vi "VI Tree.vi"   [LabVIEW 2018, in "Keithley DMM7512.lvlib"]
doc: "This is the instrument driver for the <INSTRUMENT NAME>. The VI Tree displays all the user-callable VIs of the instrument driver in an organized table."
uses:
  <instrlib>/Keithley DMM7512/Keithley DMM7512.lvlib
panel:
  # "(c) 2015 Keithley Instruments.  ALL RIGHTS RESERVED."
  # "SEE DIAGRAM\nFOR VI TREE."
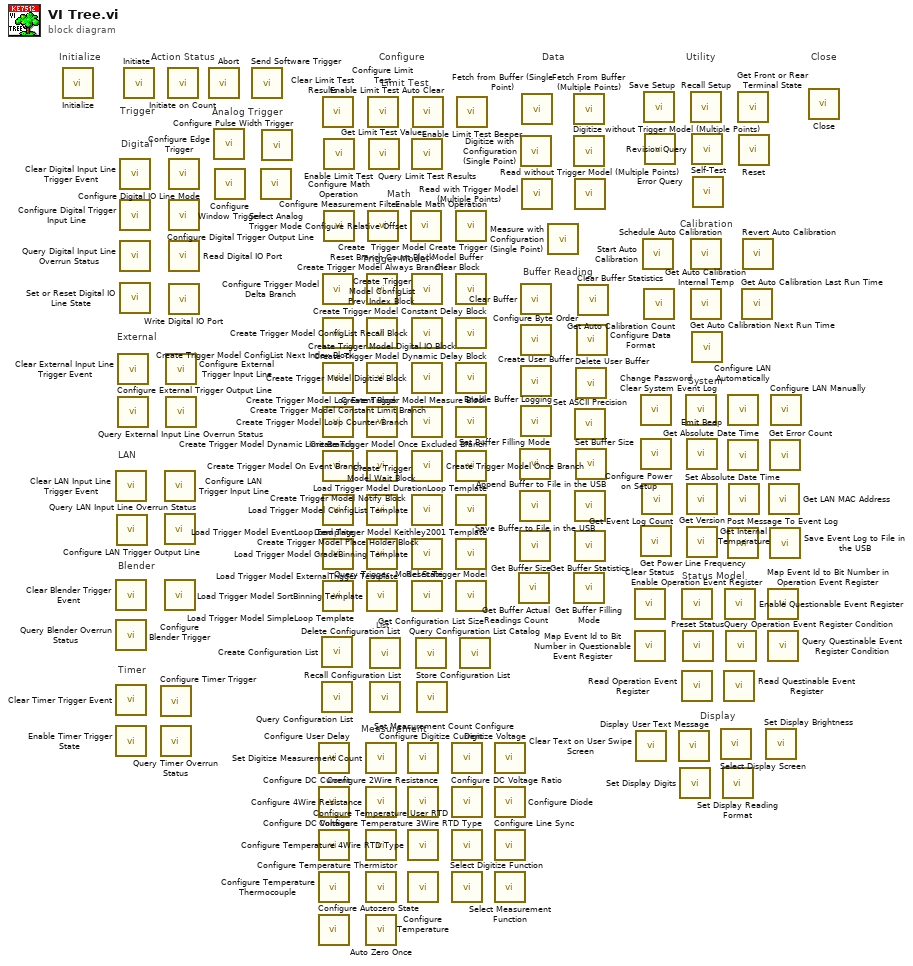
[diagram p0: block diagram]
diagram:
  # "Buffer Reading"
  # "Display"
  # "Status Model"
  # "System"
  # "Calibration"
  # "Measurement"
  # "List"
  # "Trigger Model"
  # "Math"
  # "Limit Test"
  # "Timer"
  # "Blender"
  # "LAN"
  # "External"
  # "Digital"
  # "Analog Trigger"
  # "Trigger"
  # "Action Status"
  # "Configure"
  # "Utility"
  # "Data"
  # "Close"
  # "Initialize"
  n1 = call <instrlib>:"Initialize.vi"() -> ()  [unwired: 10 in, 2 out]
  n2 = call <instrlib>:"Clear LAN Input Line Trigger Event.vi"() -> ()  [unwired: 10 in, 2 out]
  n3 = call <instrlib>:"Clear Blender Trigger Event.vi"() -> ()  [unwired: 10 in, 2 out]
  n4 = call <instrlib>:"Query Blender Overrun Status.vi"() -> ()  [unwired: 9 in, 3 out]
  n5 = call <instrlib>:"Clear Timer Trigger Event.vi"() -> ()  [unwired: 10 in, 2 out]
  n6 = call <instrlib>:"Enable Timer Trigger State.vi"() -> ()  [unwired: 14 in, 2 out]
  n7 = call <instrlib>:"Configure LAN Trigger Output Line.vi"() -> ()  [unwired: 14 in, 2 out]
  n8 = call <instrlib>:"Clear External Input Line Trigger Event.vi"() -> ()  [unwired: 10 in, 2 out]
  n9 = call <instrlib>:"Configure External Trigger Output Line.vi"() -> ()  [unwired: 10 in, 2 out]
  n10 = call <instrlib>:"Clear Digital Input Line Trigger Event.vi"() -> ()  [unwired: 10 in, 2 out]
  n11 = call <instrlib>:"Configure Digital Trigger Input Line.vi"() -> ()  [unwired: 10 in, 2 out]
  n12 = call <instrlib>:"Query Digital Input Line Overrun Status.vi"() -> ()  [unwired: 9 in, 3 out]
  n13 = call <instrlib>:"Set or Reset Digital IO Line State.vi"() -> ()  [unwired: 10 in, 2 out]
  n14 = call <instrlib>:"Initiate.vi"() -> ()  [unwired: 10 in, 2 out]
  n15 = call <instrlib>:"Configure Timer Trigger.vi"() -> ()  [unwired: 14 in, 2 out]
  n16 = call <instrlib>:"Query Timer Overrun Status.vi"() -> ()  [unwired: 9 in, 3 out]
  n17 = call <instrlib>:"Configure LAN Trigger Input Line.vi"() -> ()  [unwired: 10 in, 2 out]
  n18 = call <instrlib>:"Query LAN Input Line Overrun Status.vi"() -> ()  [unwired: 9 in, 3 out]
  n19 = call <instrlib>:"Configure Blender Trigger.vi"() -> ()  [unwired: 10 in, 2 out]
  n20 = call <instrlib>:"Configure External Trigger Input Line.vi"() -> ()  [unwired: 10 in, 2 out]
  n21 = call <instrlib>:"Query External Input Line Overrun Status.vi"() -> ()  [unwired: 9 in, 3 out]
  n22 = call <instrlib>:"Initiate on Count.vi"() -> ()  [unwired: 10 in, 2 out]
  n23 = call <instrlib>:"Configure Digital IO Line Mode.vi"() -> ()  [unwired: 10 in, 2 out]
  n24 = call <instrlib>:"Configure Digital Trigger Output Line.vi"() -> ()  [unwired: 10 in, 2 out]
  n25 = call <instrlib>:"Read Digital IO Port.vi"() -> ()  [unwired: 9 in, 3 out]
  n26 = call <instrlib>:"Write Digital IO Port.vi"() -> ()  [unwired: 10 in, 2 out]
  n27 = call <instrlib>:"Abort.vi"() -> ()  [unwired: 10 in, 2 out]
  n28 = call <instrlib>:"Configure Edge Trigger.vi"() -> ()  [unwired: 10 in, 2 out]
  n29 = call <instrlib>:"Configure Window Trigger.vi"() -> ()  [unwired: 14 in, 2 out]
  n30 = call <instrlib>:"Send Software Trigger.vi"() -> ()  [unwired: 10 in, 2 out]
  n31 = call <instrlib>:"Select Analog Trigger Mode.vi"() -> ()  [unwired: 10 in, 2 out]
  n32 = call <instrlib>:"Configure Pulse Width Trigger.vi"() -> ()  [unwired: 14 in, 2 out]
  n33 = call <instrlib>:"Configure User Delay.vi"() -> ()  [unwired: 10 in, 2 out]
  n34 = call <instrlib>:"Configure DC Current.vi"() -> ()  [unwired: 10 in, 2 out]
  n35 = call <instrlib>:"Configure DC Voltage.vi"() -> ()  [unwired: 14 in, 2 out]
  n36 = call <instrlib>:"Configure Temperature Thermocouple.vi"() -> ()  [unwired: 10 in, 2 out]
  n37 = call <instrlib>:"Configure Autozero State.vi"() -> ()  [unwired: 10 in, 2 out]
  n38 = call <instrlib>:"Create Configuration List.vi"() -> ()  [unwired: 14 in, 2 out]
  n39 = call <instrlib>:"Query Configuration List.vi"() -> ()  [unwired: 13 in, 3 out]
  n40 = call <instrlib>:"Clear Limit Test Results.vi"() -> ()  [unwired: 14 in, 2 out]
  n41 = call <instrlib>:"Configure Trigger Model Delta Branch.vi"() -> ()  [unwired: 10 in, 2 out]
  n42 = call <instrlib>:"Create Trigger Model ConfigList Next Index Block.vi"() -> ()  [unwired: 10 in, 2 out]
  n43 = call <instrlib>:"Create Trigger Model Constant Limit Branch.vi"() -> ()  [unwired: 14 in, 2 out]
  n44 = call <instrlib>:"Create Trigger Model Dynamic Limit Branch.vi"() -> ()  [unwired: 14 in, 2 out]
  n45 = call <instrlib>:"Create Trigger Model Notify Block.vi"() -> ()  [unwired: 10 in, 2 out]
  n46 = call <instrlib>:"Create Trigger Model Place Holder Block.vi"() -> ()  [unwired: 14 in, 2 out]
  n47 = call <instrlib>:"Load Trigger Model EventLoop Template.vi"() -> ()  [unwired: 14 in, 2 out]
  n48 = call <instrlib>:"Load Trigger Model SimpleLoop Template.vi"() -> ()  [unwired: 14 in, 2 out]
  n49 = call <instrlib>:"Enable Limit Test.vi"() -> ()  [unwired: 14 in, 2 out]
  n50 = call <instrlib>:"Configure Math Operation.vi"() -> ()  [unwired: 18 in, 2 out]
  n51 = call <instrlib>:"Set Digitize Measurement Count.vi"() -> ()  [unwired: 10 in, 2 out]
  n52 = call <instrlib>:"Configure 4Wire Resistance.vi"() -> ()  [unwired: 14 in, 2 out]
  n53 = call <instrlib>:"Configure Temperature User RTD.vi"() -> ()  [unwired: 10 in, 2 out]
  n54 = call <instrlib>:"Configure Temperature Thermistor.vi"() -> ()  [unwired: 10 in, 2 out]
  n55 = call <instrlib>:"Auto Zero Once.vi"() -> ()  [unwired: 10 in, 2 out]
  n56 = call <instrlib>:"Create  Trigger Model Reset Branch Count Block.vi"() -> ()  [unwired: 10 in, 2 out]
  n57 = call <instrlib>:"Create Trigger Model ConfigList Prev Index Block.vi"() -> ()  [unwired: 10 in, 2 out]
  n58 = call <instrlib>:"Create Trigger Model Digital IO Block.vi"() -> ()  [unwired: 10 in, 2 out]
  n59 = call <instrlib>:"Create Trigger Model Log Event Block.vi"() -> ()  [unwired: 10 in, 2 out]
  n60 = call <instrlib>:"Create Trigger Model On Event Branch.vi"() -> ()  [unwired: 14 in, 2 out]
  n61 = call <instrlib>:"Create Trigger Model Wait Block.vi"() -> ()  [unwired: 14 in, 2 out]
  n62 = call <instrlib>:"Load Trigger Model ExternalTrigger Template.vi"() -> ()  [unwired: 14 in, 2 out]
  n63 = call <instrlib>:"Load Trigger Model SortBinning Template.vi"() -> ()  [unwired: 26 in, 2 out]
  n64 = call <instrlib>:"Configure Limit Test.vi"() -> ()  [unwired: 14 in, 2 out]
  n65 = call <instrlib>:"Configure Measurement Filter.vi"() -> ()  [unwired: 10 in, 2 out]
  n66 = call <instrlib>:"Get Limit Test Values.vi"() -> ()  [unwired: 12 in, 4 out]
  n67 = call <instrlib>:"Delete Configuration List.vi"() -> ()  [unwired: 14 in, 2 out]
  n68 = call <instrlib>:"Recall Configuration List.vi"() -> ()  [unwired: 14 in, 2 out]
  n69 = call <instrlib>:"Set Measurement Count.vi"() -> ()  [unwired: 10 in, 2 out]
  n70 = call <instrlib>:"Configure 2Wire Resistance.vi"() -> ()  [unwired: 14 in, 2 out]
  n71 = call <instrlib>:"Configure Temperature 4Wire RTD Type.vi"() -> ()  [unwired: 10 in, 2 out]
  n72 = call <instrlib>:"Configure Temperature.vi"() -> ()  [unwired: 10 in, 2 out]
  n73 = call <instrlib>:"Configure Relative Offset.vi"() -> ()  [unwired: 10 in, 2 out]
  n74 = call <instrlib>:"Query Limit Test Results.vi"() -> ()  [unwired: 8 in, 4 out]
  n75 = call <instrlib>:"Create Trigger Model Always Branch.vi"() -> ()  [unwired: 10 in, 2 out]
  n76 = call <instrlib>:"Create Trigger Model ConfigList Recall Block.vi"() -> ()  [unwired: 10 in, 2 out]
  n77 = call <instrlib>:"Create Trigger Model Digitize Block.vi"() -> ()  [unwired: 10 in, 2 out]
  n78 = call <instrlib>:"Create Trigger Model Loop Counter Branch.vi"() -> ()  [unwired: 10 in, 2 out]
  n79 = call <instrlib>:"Create Trigger Model Once Branch.vi"() -> ()  [unwired: 10 in, 2 out]
  n80 = call <instrlib>:"Load Trigger Model ConfigList Template.vi"() -> ()  [unwired: 14 in, 2 out]
  n81 = call <instrlib>:"Load Trigger Model GradeBinning Template.vi"() -> ()  [unwired: 26 in, 2 out]
  n82 = call <instrlib>:"Query Trigger  Model State.vi"() -> ()  [unwired: 9 in, 3 out]
  n83 = call <instrlib>:"Enable Limit Test Auto Clear.vi"() -> ()  [unwired: 14 in, 2 out]
  n84 = call <instrlib>:"Get Configuration List Size.vi"() -> ()  [unwired: 13 in, 3 out]
  n85 = call <instrlib>:"Store Configuration List.vi"() -> ()  [unwired: 14 in, 2 out]
  n86 = call <instrlib>:"Configure Digitize Current.vi"() -> ()  [unwired: 14 in, 2 out]
  n87 = call <instrlib>:"Configure DC Voltage Ratio.vi"() -> ()  [unwired: 14 in, 2 out]
  n88 = call <instrlib>:"Configure Temperature 3Wire RTD Type.vi"() -> ()  [unwired: 10 in, 2 out]
  n89 = call <instrlib>:"Select Digitize Function.vi"() -> ()  [unwired: 10 in, 2 out]
  n90 = call <instrlib>:"Enable Math Operation.vi"() -> ()  [unwired: 10 in, 2 out]
  n91 = call <instrlib>:"Create Trigger Model Buffer Clear Block.vi"() -> ()  [unwired: 10 in, 2 out]
  n92 = call <instrlib>:"Create Trigger Model Constant Delay Block.vi"() -> ()  [unwired: 10 in, 2 out]
  n93 = call <instrlib>:"Create Trigger Model Dynamic Delay Block.vi"() -> ()  [unwired: 10 in, 2 out]
  n94 = call <instrlib>:"Create Trigger Model Measure Block.vi"() -> ()  [unwired: 10 in, 2 out]
  n95 = call <instrlib>:"Create Trigger Model Once Excluded Branch.vi"() -> ()  [unwired: 10 in, 2 out]
  n96 = call <instrlib>:"Load Trigger Model DurationLoop Template.vi"() -> ()  [unwired: 14 in, 2 out]
  n97 = call <instrlib>:"Load Trigger Model Keithley2001 Template.vi"() -> ()  [unwired: 14 in, 2 out]
  n98 = call <instrlib>:"Reset Trigger Model.vi"() -> ()  [unwired: 14 in, 2 out]
  n99 = call <instrlib>:"Enable Limit Test Beeper.vi"() -> ()  [unwired: 14 in, 2 out]
  n100 = call <instrlib>:"Query Configuration List Catalog.vi"() -> ()  [unwired: 13 in, 3 out]
  n101 = call <instrlib>:"Configure Digitize Voltage.vi"() -> ()  [unwired: 14 in, 2 out]
  n102 = call <instrlib>:"Configure Diode.vi"() -> ()  [unwired: 10 in, 2 out]
  n103 = call <instrlib>:"Configure Line Sync.vi"() -> ()  [unwired: 10 in, 2 out]
  n104 = call <instrlib>:"Select Measurement Function.vi"() -> ()  [unwired: 10 in, 2 out]
  n105 = call <instrlib>:"Get Buffer Actual Readings Count.vi"() -> ()  [unwired: 13 in, 3 out]
  n106 = call <instrlib>:"Set Buffer Filling Mode.vi"() -> ()  [unwired: 14 in, 2 out]
  n107 = call <instrlib>:"Save Buffer to File in the USB.vi"() -> ()  [unwired: 14 in, 2 out]
  n108 = call <instrlib>:"Get Buffer Size.vi"() -> ()  [unwired: 13 in, 3 out]
  n109 = call <instrlib>:"Digitize with Configuration (Single Point).vi"() -> ()  [unwired: 8 in, 4 out]
  n110 = call <instrlib>:"Clear Buffer.vi"() -> ()  [unwired: 14 in, 2 out]
  n111 = call <instrlib>:"Configure Byte Order.vi"() -> ()  [unwired: 14 in, 2 out]
  n112 = call <instrlib>:"Create User Buffer.vi"() -> ()  [unwired: 14 in, 2 out]
  n113 = call <instrlib>:"Enable Buffer Logging.vi"() -> ()  [unwired: 10 in, 2 out]
  n114 = call <instrlib>:"Fetch from Buffer (Single Point).vi"() -> ()  [unwired: 8 in, 4 out]
  n115 = call <instrlib>:"Read with Trigger Model (Multiple Points).vi"() -> ()  [unwired: 8 in, 4 out]
  n116 = call <instrlib>:"Measure with Configuration (Single Point).vi"() -> ()  [unwired: 8 in, 4 out]
  n117 = call <instrlib>:"Fetch From Buffer (Multiple Points).vi"() -> ()  [unwired: 8 in, 4 out]
  n118 = call <instrlib>:"Digitize without Trigger Model (Multiple Points).vi"() -> ()  [unwired: 8 in, 4 out]
  n119 = call <instrlib>:"Get Buffer Filling Mode.vi"() -> ()  [unwired: 13 in, 3 out]
  n120 = call <instrlib>:"Read without Trigger Model (Multiple Points).vi"() -> ()  [unwired: 8 in, 4 out]
  n121 = call <instrlib>:"Set ASCII Precision.vi"() -> ()  [unwired: 14 in, 2 out]
  n122 = call <instrlib>:"Append Buffer to File in the USB.vi"() -> ()  [unwired: 14 in, 2 out]
  n123 = call <instrlib>:"Get Buffer Statistics.vi"() -> ()  [unwired: 13 in, 3 out]
  n124 = call <instrlib>:"Delete User Buffer.vi"() -> ()  [unwired: 14 in, 2 out]
  n125 = call <instrlib>:"Set Buffer Size.vi"() -> ()  [unwired: 14 in, 2 out]
  n126 = call <instrlib>:"Configure Data Format.vi"() -> ()  [unwired: 14 in, 2 out]
  n127 = call <instrlib>:"Clear Buffer Statistics.vi"() -> ()  [unwired: 14 in, 2 out]
  n128 = call <instrlib>:"Clear Status.vi"() -> ()  [unwired: 10 in, 2 out]
  n129 = call <instrlib>:"Map Event Id to Bit Number in Questionable Event Register.vi"() -> ()  [unwired: 10 in, 2 out]
  n130 = call <instrlib>:"Clear Text on User Swipe Screen.vi"() -> ()  [unwired: 10 in, 2 out]
  n131 = call <instrlib>:"Change Password.vi"() -> ()  [unwired: 10 in, 2 out]
  n132 = call <instrlib>:"Configure Power on Setup.vi"() -> ()  [unwired: 10 in, 2 out]
  n133 = call <instrlib>:"Get Power Line Frequency.vi"() -> ()  [unwired: 9 in, 3 out]
  n134 = call <instrlib>:"Get Event Log Count.vi"() -> ()  [unwired: 9 in, 3 out]
  n135 = call <instrlib>:"Start Auto Calibration.vi"() -> ()  [unwired: 10 in, 2 out]
  n136 = call <instrlib>:"Save Setup.vi"() -> ()  [unwired: 10 in, 2 out]
  n137 = call <instrlib>:"Get Auto Calibration Count.vi"() -> ()  [unwired: 9 in, 3 out]
  n138 = call <instrlib>:"Error Query.vi"() -> ()  [unwired: 8 in, 4 out]
  n139 = call <instrlib>:"Display User Text Message.vi"() -> ()  [unwired: 10 in, 2 out]
  n140 = call <instrlib>:"Set Display Digits.vi"() -> ()  [unwired: 10 in, 2 out]
  n141 = call <instrlib>:"Enable Operation Event Register.vi"() -> ()  [unwired: 10 in, 2 out]
  n142 = call <instrlib>:"Read Operation Event Register.vi"() -> ()  [unwired: 9 in, 3 out]
  n143 = call <instrlib>:"Preset Status.vi"() -> ()  [unwired: 10 in, 2 out]
  n144 = call <instrlib>:"Clear System Event Log.vi"() -> ()  [unwired: 10 in, 2 out]
  n145 = call <instrlib>:"Emit Beep.vi"() -> ()  [unwired: 10 in, 2 out]
  n146 = call <instrlib>:"Set Absolute Date Time.vi"() -> ()  [unwired: 14 in, 2 out]
  n147 = call <instrlib>:"Get Version.vi"() -> ()  [unwired: 9 in, 3 out]
  n148 = call <instrlib>:"Recall Setup.vi"() -> ()  [unwired: 10 in, 2 out]
  n149 = call <instrlib>:"Schedule Auto Calibration.vi"() -> ()  [unwired: 10 in, 2 out]
  n150 = call <instrlib>:"Get Auto Calibration Internal Temp.vi"() -> ()  [unwired: 9 in, 3 out]
  n151 = call <instrlib>:"Revision Query.vi"() -> ()  [unwired: 8 in, 4 out]
  n152 = call <instrlib>:"Get Auto Calibration Next Run Time.vi"() -> ()  [unwired: 9 in, 3 out]
  n153 = call <instrlib>:"Self-Test.vi"() -> ()  [unwired: 8 in, 4 out]
  n154 = call <instrlib>:"Select Display Screen.vi"() -> ()  [unwired: 10 in, 2 out]
  n155 = call <instrlib>:"Set Display Reading Format.vi"() -> ()  [unwired: 14 in, 2 out]
  n156 = call <instrlib>:"Read Questinable Event Register.vi"() -> ()  [unwired: 9 in, 3 out]
  n157 = call <instrlib>:"Enable Questionable Event Register.vi"() -> ()  [unwired: 10 in, 2 out]
  n158 = call <instrlib>:"Query Operation Event Register Condition.vi"() -> ()  [unwired: 9 in, 3 out]
  n159 = call <instrlib>:"Configure LAN Automatically.vi"() -> ()  [unwired: 10 in, 2 out]
  n160 = call <instrlib>:"Get Absolute Date Time.vi"() -> ()  [unwired: 8 in, 8 out]
  n161 = call <instrlib>:"Post Message To Event Log.vi"() -> ()  [unwired: 10 in, 2 out]
  n162 = call <instrlib>:"Get Internal Temperature.vi"() -> ()  [unwired: 9 in, 3 out]
  n163 = call <instrlib>:"Get Front or Rear Terminal State.vi"() -> ()  [unwired: 9 in, 3 out]
  n164 = call <instrlib>:"Reset.vi"() -> ()  [unwired: 10 in, 2 out]
  n165 = call <instrlib>:"Get Auto Calibration Last Run Time.vi"() -> ()  [unwired: 9 in, 3 out]
  n166 = call <instrlib>:"Revert Auto Calibration.vi"() -> ()  [unwired: 10 in, 2 out]
  n167 = call <instrlib>:"Set Display Brightness.vi"() -> ()  [unwired: 10 in, 2 out]
  n168 = call <instrlib>:"Map Event Id to Bit Number in Operation Event Register.vi"() -> ()  [unwired: 10 in, 2 out]
  n169 = call <instrlib>:"Query Questinable Event Register Condition.vi"() -> ()  [unwired: 9 in, 3 out]
  n170 = call <instrlib>:"Get LAN MAC Address.vi"() -> ()  [unwired: 9 in, 3 out]
  n171 = call <instrlib>:"Get Error Count.vi"() -> ()  [unwired: 9 in, 3 out]
  n172 = call <instrlib>:"Save Event Log to File in the USB.vi"() -> ()  [unwired: 10 in, 2 out]
  n173 = call <instrlib>:"Configure LAN Manually.vi"() -> ()  [unwired: 10 in, 2 out]
  n174 = call <instrlib>:"Close.vi"() -> ()  [unwired: 11 in, 1 out]
